vi "UI_Device_Lubricate_Unit_Test2.vi"() -> ()   [LabVIEW 2014]
panel:
  in  "陪试轴承单元供油过滤器1堵塞":bool caption="供油过滤器1堵塞"
  in  "陪试轴承单元油箱液位过低":bool caption="油箱液位过低"
  in  "陪试轴承单元油箱液位过高":bool caption="油箱液位过高"
  in  "陪试轴承单元回油过滤器堵塞":bool caption="回油过滤器堵塞"
  in  "陪试轴承单元供油过滤器2堵塞":bool caption="供油过滤器2堵塞"
  out "传感器出油温度2":dbl
  out "传感器出油温度1":dbl
  in  "退出":bool
  out "低压供油压力":dbl(graph)
  out "供油温度":dbl(graph)
  out "供油流量":dbl(graph)
  out "陪试轴承单元调试状态":bool
  in  "开始调试":bool
  # "陪试轴承单元独立调试"
  # "监测参数"
  # "传\n感\n器"
  # "报警信息"
  # "单\n元\n系\n统"
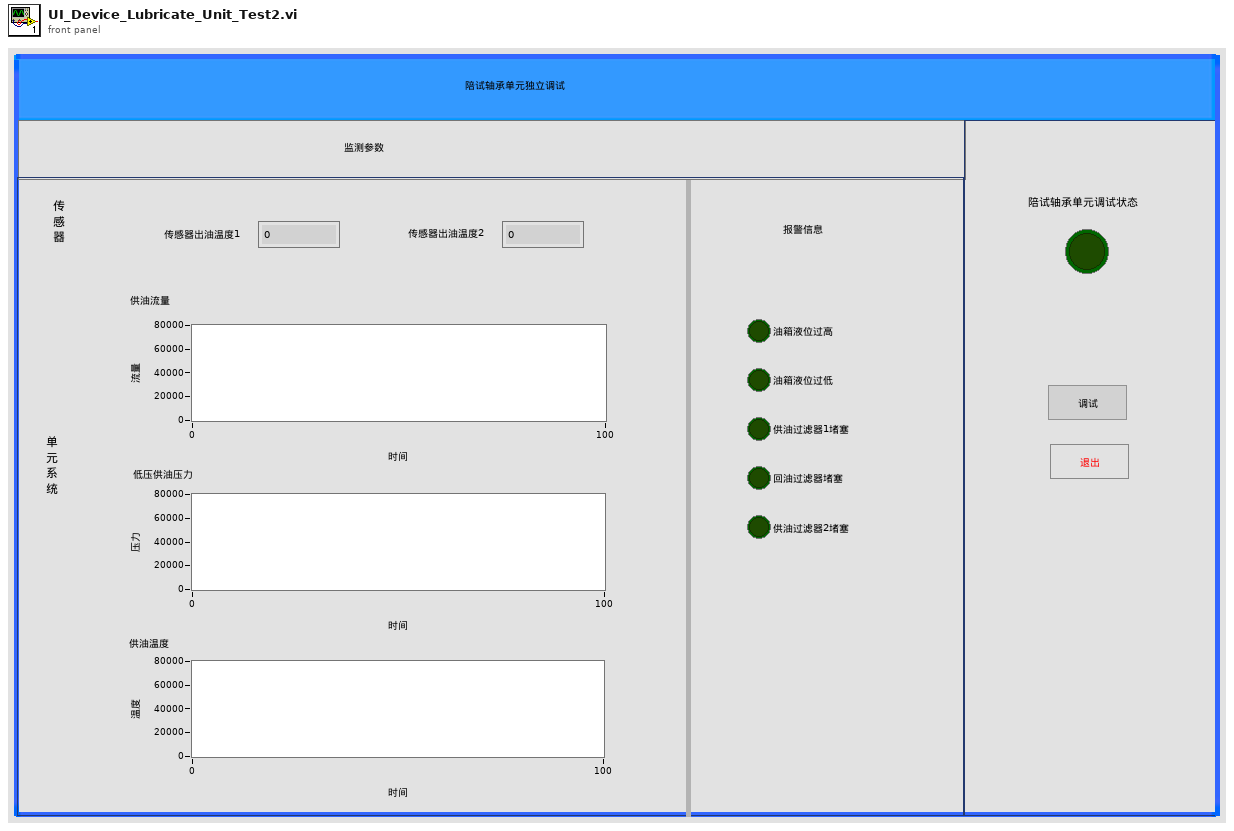
[diagram p1: front panel]
types:
  T1 = cluster{"径向油缸加载压力":u16, "轴向油缸加载压力":u16, "油箱1油液温度":u16, "润滑油温度":u16, "油箱2油液温度":u16, "试验轴承供油压力":u16, "试验轴承供油流量":u16, "陪试轴承供油流量":u16, "陪试轴承供油压力":u16, "陪试轴承供油温度":u16, "液压子系统状态字":cluster{"加载单元":cluster{"供油过滤器堵塞报警":bool, "回油过滤器堵塞报警":bool, "液位过高报警":bool, "液位过低报警":bool}, "试验轴承单元":cluster{"加热装置异常报警":bool, "油箱1液位过高报警":bool, "油箱1液位过低报警":bool, "油箱2液位过高报警":bool, "油箱2液位过低报警":bool, "供油过滤器堵塞报警":bool, "循环回路过滤器堵塞报警":bool, "回油过滤器堵塞报警":bool}, "陪试轴承单元":cluster{"供油过滤器1堵塞报警":bool, "供油过滤器2堵塞报警":bool, "回油过滤器堵塞报警":bool, "油箱液位过高报警":bool, "油箱液位过低报警":bool}}}
  T2 = cluster{"时间":timestamp, "陪试轴承润滑单元出油温度1":sgl[], "陪试轴承润滑单元出油温度2":sgl[], "轴承外圈温度":sgl[], "出油温度":sgl[], "摩擦力1":sgl[], "摩擦力2":sgl[], "径向油缸力":sgl[], "轴向油缸力":sgl[], "转速":sgl[]}
  T3 = cluster{"供油过滤器1堵塞报警":bool, "供油过滤器2堵塞报警":bool, "回油过滤器堵塞报警":bool, "油箱液位过高报警":bool, "油箱液位过低报警":bool}
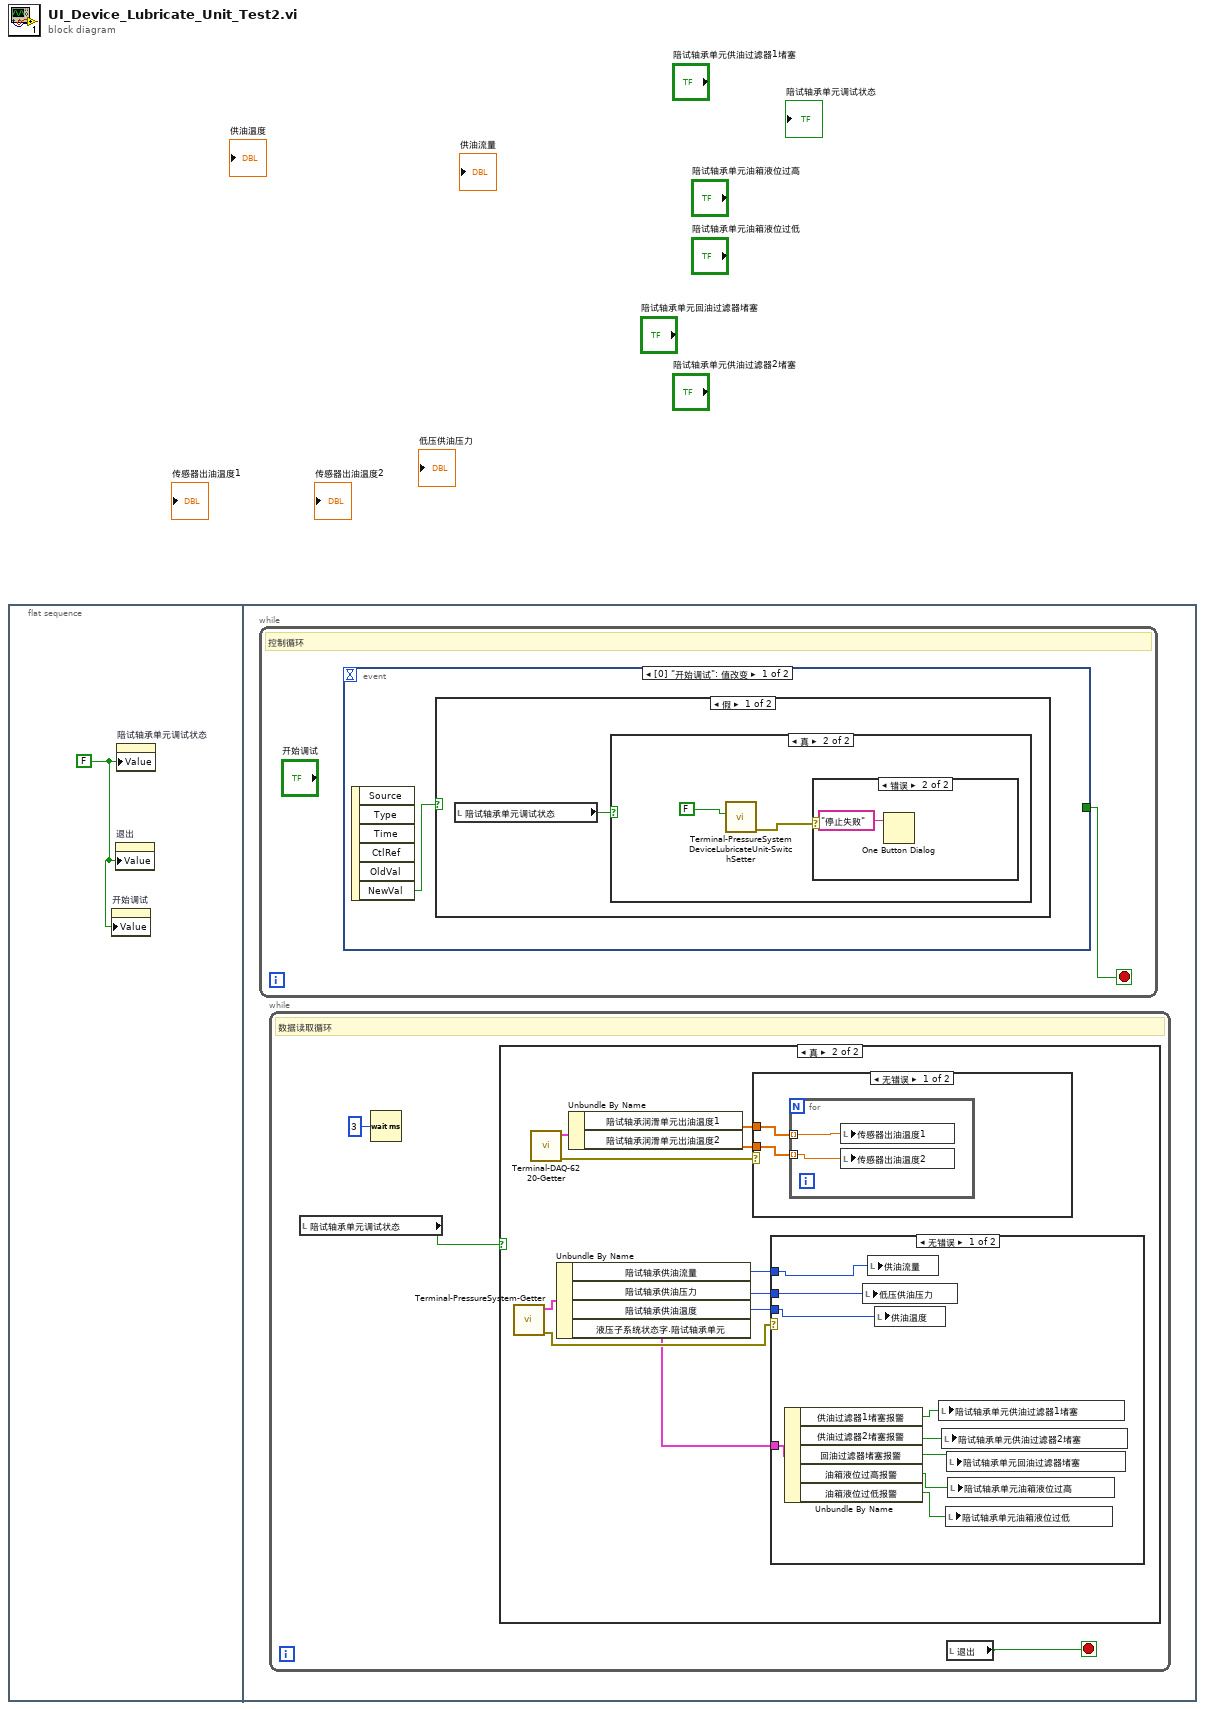
[diagram p0: block diagram]
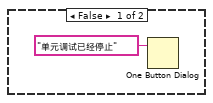
[diagram p5: hidden frame]
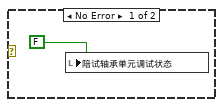
[diagram p6: hidden frame]
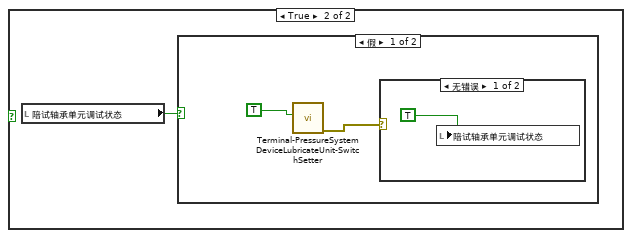
[diagram p7: hidden frame]
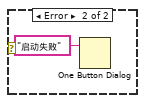
[diagram p8: hidden frame]
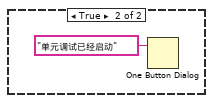
[diagram p9: hidden frame]
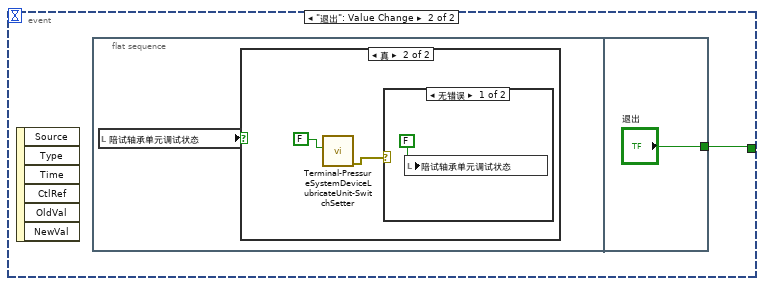
[diagram p10: hidden frame]
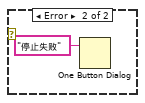
[diagram p12: hidden frame]
diagram:
  n1 = flat-sequence {
    frame #0 {
      w1 = FALSE ("陪试轴承单元调试状态")
      n2 = property on="开始调试" class="Bool (严格)"("Value"=w1) -> ()  [unwired: 2 in, 2 out]
      n3 = property on="退出" class="Bool (严格)"("Value"=w1) -> ()  [unwired: 2 in, 2 out]
      n4 = property on="陪试轴承单元调试状态" class="Bool (严格)"("Value"=w1) -> ()  [unwired: 2 in, 2 out]
    }
    frame #1 {
      n5 = while {
        stop <- w28 stop-if-true
        # "控制循环"
        n6 = event shown="[0] \"开始调试\": 值改变" {
          selector: _ -> [_ _]
          dyn-events: _ -> [_ _]
          timeout: _ -> [_ _]
          tunnel: [_ w42] -> w28
          event "开始调试": Value Change {
            n7 = event-data() -> ("NewVal"=w29:bool)  [unwired: 1 in, 5 out]
            n8 = case shown="假" w29 {
              frame False {
                n9 = local read "陪试轴承单元调试状态"() -> (w30:bool)
                n10 = case shown="真" w30 {
                  frame False {
                    n11 = One Button Dialog(message="单元调试已经停止" ("消息")) -> ()  [unwired: 1 in, 1 out]
                  }
                  frame True {
                    n12 = call "Terminal-PressureSystemDeviceLubricateUnit-SwitchSetter.vi"("启停"=FALSE) -> ("error out"=w33:errorcluster)  [unwired: 10 in]
                    n13 = case shown="错误" w33 {
                      frame No Error {
                        n14 = local write "陪试轴承单元调试状态"(FALSE) -> ()
                      }
                      frame Error {
                        n15 = One Button Dialog(message="停止失败" ("消息")) -> ()  [unwired: 1 in, 1 out]
                      }
                    }
                  }
                }
              }
              frame True {
                n16 = local read "陪试轴承单元调试状态"() -> (w36:bool)
                n17 = case shown="假" w36 {
                  frame False {
                    n18 = call "Terminal-PressureSystemDeviceLubricateUnit-SwitchSetter.vi"("启停"=TRUE) -> ("error out"=w38:errorcluster)  [unwired: 10 in]
                    n19 = case shown="无错误" w38 {
                      frame No Error {
                        n20 = local write "陪试轴承单元调试状态"(TRUE) -> ()
                      }
                      frame Error {
                        n21 = One Button Dialog(message="启动失败" ("消息")) -> ()  [unwired: 1 in, 1 out]
                      }
                    }
                  }
                  frame True {
                    n22 = One Button Dialog(message="单元调试已经启动" ("消息")) -> ()  [unwired: 1 in, 1 out]
                  }
                }
              }
            }
          }
          event "退出": Value Change {
            n23 = event-data() -> ()  [unwired: 1 in, 6 out]
            n24 = flat-sequence {
              tunnel: ["退出"] -> w42
              frame #0 {
                n25 = local read "陪试轴承单元调试状态"() -> (w43:bool)
                n26 = case shown="真" w43 {
                  frame False {
                  }
                  frame True {
                    n27 = call "Terminal-PressureSystemDeviceLubricateUnit-SwitchSetter.vi"("启停"=FALSE) -> ("error out"=w45:errorcluster)  [unwired: 10 in]
                    n28 = case shown="无错误" w45 {
                      frame No Error {
                        n29 = local write "陪试轴承单元调试状态"(FALSE) -> ()
                      }
                      frame Error {
                        n30 = One Button Dialog(message="停止失败" ("消息")) -> ()  [unwired: 1 in, 1 out]
                      }
                    }
                  }
                }
              }
              frame #1 {
              }
            }
          }
        }
      }
      n31 = while {
        stop <- w3 stop-if-true
        # "数据读取循环"
        n32 = local read "陪试轴承单元调试状态"() -> (w4:bool)
        n33 = Wait (ms)(milliseconds to wait=u32 3 ("等待时间（毫秒）")) -> ()  [unwired: 1 out]
        n34 = case shown="真" w4 {
          frame False {
          }
          frame True {
            n35 = call "Terminal-PressureSystem-Getter.vi"() -> ("error out"=w10:errorcluster, "设备信息"=w9:T1)  [unwired: 10 in]
            n36 = call "Terminal-DAQ-6220-Getter.vi"() -> ("error out"=w14:errorcluster, "6220"=w13:T2)  [unwired: 10 in]
            n37 = Unbundle By Name(w9) -> ("陪试轴承供油流量"=w7:u16, "陪试轴承供油压力"=w5:u16, "陪试轴承供油温度"=w6:u16, "液压子系统状态字.陪试轴承单元"=w8:T3)
            n38 = Unbundle By Name(w13) -> ("陪试轴承润滑单元出油温度1"=w12:sgl[], "陪试轴承润滑单元出油温度2"=w11:sgl[])
            n39 = case shown="无错误" w14 {
              tunnel: w12 -> [w25 _]
              tunnel: w11 -> [w24 _]
              frame No Error {
                n40 = for {
                  tunnel: w25 -> [w27] mode=indexing
                  tunnel: w24 -> [w26] mode=indexing
                  n41 = local write "传感器出油温度1"(w27) -> ()
                  n42 = local write "传感器出油温度2"(w26) -> ()
                }
              }
              frame Error {
              }
            }
            n43 = case shown="无错误" w10 {
              tunnel: w8 -> [w23 _]
              tunnel: w7 -> [w15 _]
              tunnel: w6 -> [w18 _]
              tunnel: w5 -> [w17 _]
              frame No Error {
                n44 = Unbundle By Name(w23) -> ("供油过滤器1堵塞报警"=w22:bool, "供油过滤器2堵塞报警"=w21:bool, "回油过滤器堵塞报警"=w20:bool, "油箱液位过高报警"=w19:bool, "油箱液位过低报警"=w16:bool)
                n45 = local write "低压供油压力"(w17) -> ()
                n46 = local write "供油流量"(w15) -> ()
                n47 = local write "供油温度"(w18) -> ()
                n48 = local write "陪试轴承单元供油过滤器1堵塞"(w22) -> ()
                n49 = local write "陪试轴承单元供油过滤器2堵塞"(w21) -> ()
                n50 = local write "陪试轴承单元油箱液位过低"(w16) -> ()
                n51 = local write "陪试轴承单元回油过滤器堵塞"(w20) -> ()
                n52 = local write "陪试轴承单元油箱液位过高"(w19) -> ()
              }
              frame Error {
              }
            }
          }
        }
        n53 = local read "退出"() -> (w3:bool)
      }
    }
  }
